vi "File writer.vi"() -> ()   [LabVIEW 2018]
panel:
  out "path":path
  out "Combinada":string
  in  "#1":dbl
  in  "#2":dbl
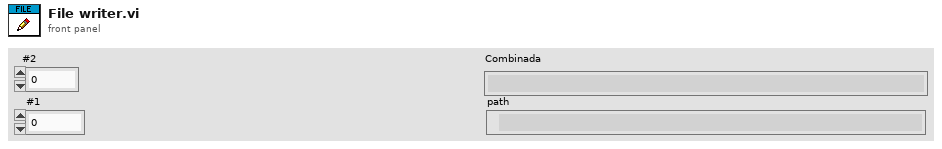
[diagram p1: front panel]
types:
  T1 = enum16{"open", "replace", "create", "open or create", "replace or create", "replace or create with confirmation"}
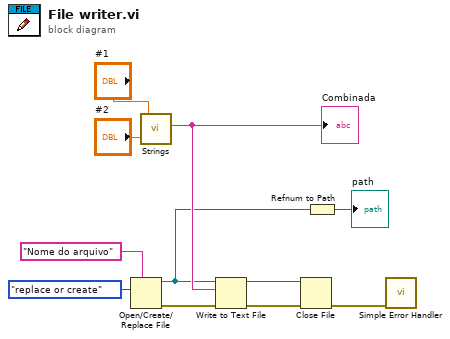
[diagram p0: block diagram]
diagram:
  n1 = Open/Create/Replace File(prompt="Nome do arquivo", operation (0:open)=T1."replace or create") -> (refnum out=w2:refnum<file>, error out=w10:errorcluster)  [unwired: 4 in, 1 out]
  n2 = call "Strings.vi"("#2"="#2", "#1"="#1") -> ("Combinada"=w3:string)
  "Combinada" <- w3
  n3 = Write to Text File(file (use dialog)=w2, text=w3, error in=w10) -> (refnum out=w11:refnum<file>, error out=w9:errorcluster)  [unwired: 1 in, 1 out]
  n4 = Close File(refnum=w11, error in=w9) -> (error out=w8:errorcluster)  [unwired: 1 out]
  n5 = Refnum to Path(1:w2) -> (0:→"path":path)
  n6 = call <vilib>:"Simple Error Handler.vi"("error in (no error)"=w8) -> ()  [unwired: 4 in, 5 out]
